vi "choose firs acquisition state.vi"(8 "error in (no error)":errorcluster, 11 "Channel in":refnum<class "ECHARPE_Channel.lvclass">) -> (0 "error out":errorcluster, 2 "verify S4ICS status":bool, 3 "Channel out":refnum<class "ECHARPE_Channel.lvclass">)   [LabVIEW 2018, in "ECHARPE_Channel.lvclass"]
uses:
  ECHARPE_Channel.lvclass
  Server/Server.lvclass/Server.ctl
  RxTx/RxTx.lvclass
  Server/Server.lvclass
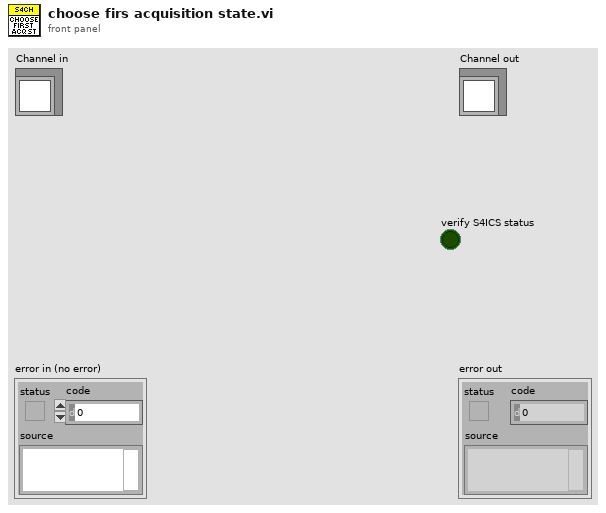
[diagram p1: front panel]
types:
  T1 = cluster{"State Machine.lvclass":refnum<class "State Machine.lvclass">, "RxTx.lvclass":refnum<class "RxTx.lvclass">, "Save_Header_RxTx.lvclass":refnum<class "RxTx.lvclass">, "Status SM.lvclass":refnum<class "State Machine.lvclass">, "Status RxTx.lvclass":refnum<class "RxTx.lvclass">, "servers array":refnum<class "Server.lvclass">[], "Events log file.lvclass":refnum<class "Log File.lvclass">, "Errors log file.lvclass":refnum<class "Log File.lvclass">, "Keywords log file.lvclass":refnum<class "Log File.lvclass">, "Sim_CCD.lvclass":refnum<class "Sim_CCD.lvclass">}
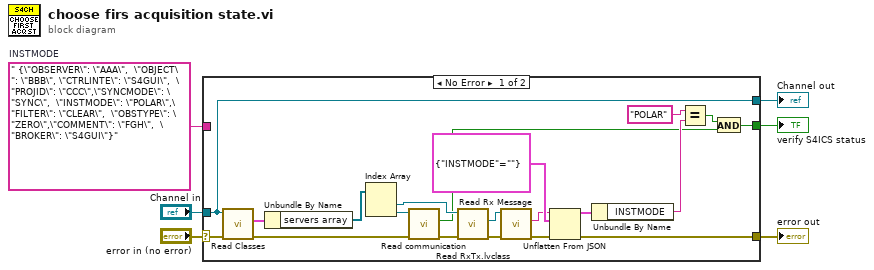
[diagram p0: block diagram]
diagram:
  w2 = " {\"OBSERVER\": \"AAA\",  \"OBJECT\": \"BBB\", \"CTRLINTE\": \"S4GUI\",  \"PROJID\": \"CCC\",\"SYNCMODE\": \"SYNC\",  \"INSTMODE\": \"POLAR\",\"FILTER\": \"CLEAR\",  \"OBSTYPE\": \"ZERO\",\"COMMENT\": \"FGH\",  \"BROKER\": \"S4GUI\"}"  # INSTMODE
  n1 = case shown="No Error" "error in (no error)" {
    selector: "error in (no error)" -> [w8 w28]
    tunnel: [w21 w28] -> w5
    tunnel: [w9 w27] -> w3
    tunnel: "Channel in" -> [w9 w27]
    tunnel: w2 -> [_ _]
    tunnel: [w12 _] -> w1
    frame No Error {
      n2 = call-dynamic "Read Classes.vi"("error in (no error)"=w8, "Channel in"=w9) -> ("error out"=w7:errorcluster, "Classes"=w10:T1)  [unwired: 7 in, 1 out]
      n3 = Unbundle By Name(w10) -> ("servers array"=w11:refnum<class "Server.lvclass">[])
      n4 = Index Array(array=w11) -> (element #1=w17:refnum<class "Server.lvclass">, element #2=w16:refnum<class "Server.lvclass">)  [unwired: 2 in]
      n5 = call "Read communication.vi"("error in (no error)"=w7, "Server in"=w16) -> ("error out"=w15:errorcluster, "communication"=w13:bool)  [unwired: 7 in, 1 out]
      n6 = call "Read RxTx.lvclass.vi"("error in (no error)"=w15, "Server in"=w17) -> ("error out"=w25:errorcluster, "RxTx.lvclass"=w26:refnum<class "RxTx.lvclass">)  [unwired: 7 in, 1 out]
      n7 = call "Read Rx Message.vi"("error in (no error)"=w25, "RxTx in"=w26) -> ("error out"=w24:errorcluster, "Rx Message"=w14:string)  [unwired: 7 in, 1 out]
      n8 = Unflatten From JSON(JSON string=w14, type and defaults=cluster{"INSTMODE":string} {"INSTMODE"=""}, error in (no error)=w24) -> (value=w23:cluster{"INSTMODE":string}, error out=w21:errorcluster)  [unwired: 4 in]
      n9 = Unbundle By Name(w23) -> ("INSTMODE"=w20:string)
      n10 = Equal?(x="POLAR", y=w20) -> (x = y?=w18:bool)
      n11 = And(x=w18, y=w13) -> (x .and. y?=w12:bool)
    }
    frame Error {
    }
  }
  "error out" <- w5
  "Channel out" <- w3
  "verify S4ICS status" <- w1
